vi "Add Error Group.vi"(8 "error in (no error)":errorcluster, 11 "Parent Ref in":T1 format="%.0x") -> (0 "error out":errorcluster, 3 "Parent Ref out":T1 format="%.0x")   [LabVIEW 2021, in "Modbus Master System Explorer.lvlib"]
uses:
  Modbus Master System Explorer.lvlib
  <vilib>/NI VeriStand/Custom Device API/Custom Device Item Ref.ctl
  <vilib>/NI VeriStand/Custom Device API/Custom Device Channel.ctl
  <vilib>/NI VeriStand/Custom Device API/Custom Device Channel Type.ctl
  Shared/Constants.vi
  <vilib>/NI VeriStand/Custom Device API/Custom Device API.lvlib
  Shared/Modbus Master Shared.lvlib
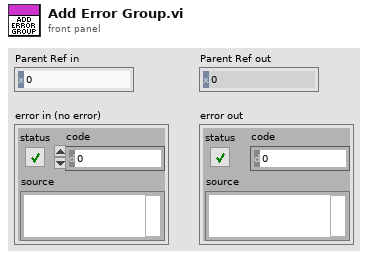
[diagram p1: front panel]
types:
  T1 = typedef "Custom Device API.lvlib/Custom Device Item Ref.ctl" = u64
  T2 = typedef "Custom Device API.lvlib/Custom Device Channel.ctl" = cluster{"Type":T3, "Units":string, "Default Value":dbl, "Faultable":bool, "Scalable":bool}
  T3 = typedef "Custom Device API.lvlib/Custom Device Channel Type.ctl" = enum16{"Input", "Output"}
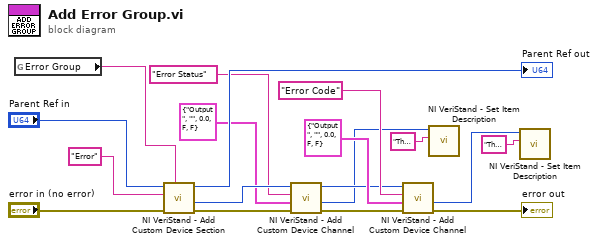
[diagram p0: block diagram]
diagram:
  n1 = global read "Constants.vi" "Error Group"() -> (w5:string)
  n2 = call <vilib>:"NI VeriStand - Add Custom Device Section.vi"("GUID (Default Section)"=w5, "error in (no error)"="error in (no error)", "Section Name"="Error", "Parent Ref in"="Parent Ref in") -> ("error out"=w17:errorcluster, "Section Ptr"=w15:T1, "Parent Ref out"=→"Parent Ref out":T1)  [unwired: 4 in, 1 out]
  n3 = call <vilib>:"NI VeriStand - Add Custom Device Channel.vi"("error in (no error)"=w17, "Channel"=T2 {"Type"=enum."Output", "Units"="", "Default Value"=0.0, "Faultable"=FALSE, "Scalable"=FALSE}, "Channel Name"="Error Status", "Parent Ref in"=w15) -> ("error out"=w8:errorcluster, "Channel Ref"=w4:T1, "Parent Ref out"=w9:T1)  [unwired: 4 in, 1 out]
  n4 = call <vilib>:"NI VeriStand - Add Custom Device Channel.vi"("error in (no error)"=w8, "Channel"=T2 {"Type"=enum."Output", "Units"="", "Default Value"=0.0, "Faultable"=FALSE, "Scalable"=FALSE}, "Channel Name"="Error Code", "Parent Ref in"=w9) -> ("error out"=→"error out":errorcluster, "Channel Ref"=w2:T1)  [unwired: 4 in, 2 out]
  n5 = call <vilib>:"NI VeriStand - Set Item Description.vi"("Description"="The Error Status channel is toggled in the event that a LabVIEW error other than a network timeout occurs. ", "Item Ref in"=w4) -> ()  [unwired: 7 in, 3 out]
  n6 = call <vilib>:"NI VeriStand - Set Item Description.vi"("Description"="The Error Code channel reports any LabVIEW errors that occur in the engine at runtime. Because Error 56 (Network Timeout) is non-critical in this application, it is cleared and the Timeout? channel is toggled instead.", "Item Ref in"=w2) -> ()  [unwired: 7 in, 3 out]
